vi "Call(Dynamic).vi"(8 "error in (no error)":errorcluster) -> (0 "error out":errorcluster)   [LabVIEW 2019, in "Camera Engine.lvlib"]
uses:
  Camera Engine.lvlib
  <userlib>/JUL/Common Module/Com Library/Com SubVI/Com_SubVI_Call Dynamic VI(Hide).vi
  <userlib>/JUL/Common Module/Com Library/Common.lvlib
panel:
  # "Input"
  # "Output"
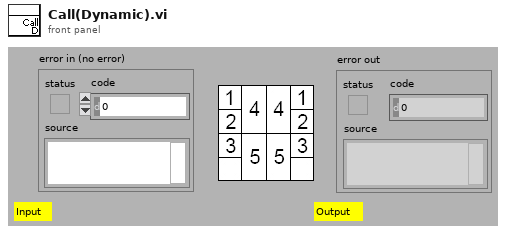
[diagram p1: front panel]
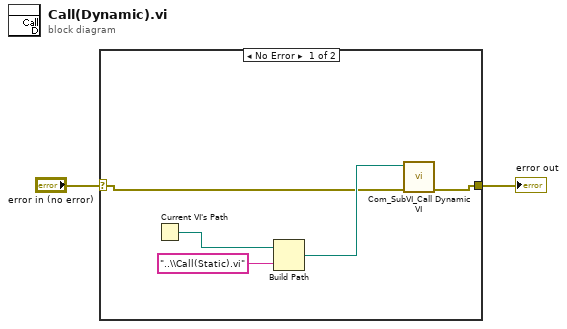
[diagram p0: block diagram]
diagram:
  n1 = case shown="No Error" "error in (no error)" {
    selector: "error in (no error)" -> [w4 w8]
    tunnel: [w3 w8] -> w1
    frame No Error {
      n2 = Current VI's Path() -> (path=w7:path)
      n3 = Build Path(base path=w7, name or relative path="..\\Call(Static).vi") -> (appended path=w5:path)
      n4 = call-poly <userlib>:"Com_SubVI_Call Dynamic VI.vi"("error in (no error)"=w4, "Path"=w5) -> ("error out"=w3:errorcluster)  [unwired: 9 in]
    }
    frame Error {
    }
  }
  "error out" <- w1
